vi "Get Control Refnum from Label.vi"(8 "error in (no error)":errorcluster, 9 "search field":enum16{"label", "caption", "label & caption"}(ring)=enum."label & caption", 10 "Control name":string, 11 "VI reference":refnum<vi>) -> (0 "error out":errorcluster, 1 "found?":bool, 2 "Ctl Refnum":refnum<vi>, 3 "VI reference out":refnum<vi>)   [LabVIEW 2009]
doc: "Takes a string and a reference to a VI, and searches all controls on the front panel of that VI for a control with a label that matches the input string, a label that does, or either one matches. Returns a reference to the first matching control found, or an empty reference if no controls matched."
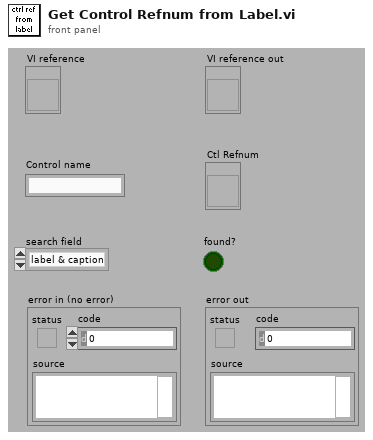
[diagram p1: front panel]
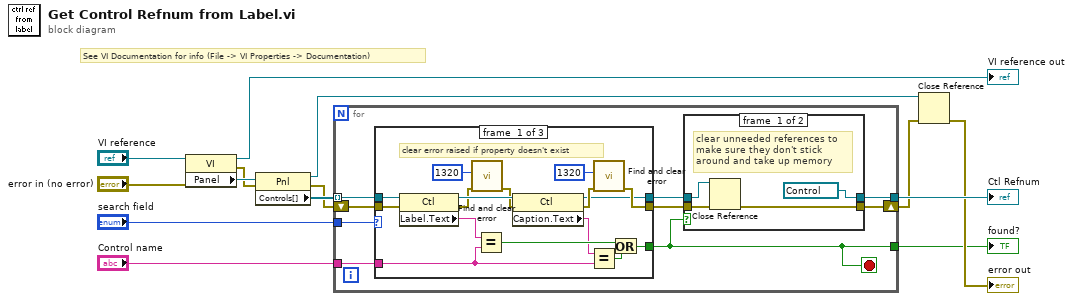
[diagram p0: block diagram]
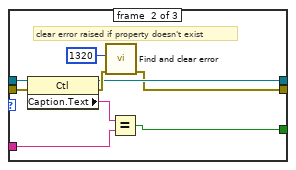
[diagram p2: hidden frame]
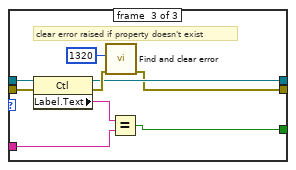
[diagram p3: hidden frame]
diagram:
  # "See VI Documentation for info (File -> VI Properties -> Documentation)"
  n1 = property class="VI"(reference="VI reference", error in="error in (no error)") -> (reference out=→"VI reference out":refnum<vi>, error out=w10:errorcluster, "Panel"=w13:refnum<vi>)
  n2 = property class="Pnl"(reference=w13, error in=w10) -> (reference out=w6:refnum<vi>, error out=w9:errorcluster, "Controls[]"=w12:refnum<vi>[])
  n3 = for {
    tunnel: w12 -> [w23] mode=indexing
    tunnel: "Control name" -> [w17]
    tunnel: [w15] -> w2
    shift-right: [w20] -> w5
    shift-left: w9 -> [w19]
    tunnel: [w18] -> w7
    tunnel: "search field" -> [w16]
    stop <- w15 stop-if-true
    n4 = case shown="\"label & caption\"" w16 {
      tunnel: w23 -> [w39 w48 w57]
      tunnel: [w27 w42 w51] -> w22
      tunnel: [w29 w41 w50] -> w21
      tunnel: w19 -> [w38 w47 w56]
      tunnel: w17 -> [w25 w43 w52]
      tunnel: [w35 w40 w49] -> w15
      frame #0 {
        # "clear error raised if property doesn't exist"
        n5 = property class="Ctl"(reference=w39, error in=w38) -> (reference out=w33:refnum<vi>, error out=w32:errorcluster, "Label.Text"=w37:string)
        n6 = call "Find and clear error.vi"("error in (no error)"=w32, "error code"=1320) -> ("error out"=w31:errorcluster)  [unwired: 9 out]
        n7 = Equal?(x=w37, y=w25) -> (x = y?=w36:bool)
        n8 = property class="Ctl"(reference=w33, error in=w31) -> (reference out=w27:refnum<vi>, error out=w28:errorcluster, "Caption.Text"=w26:string)
        n9 = Equal?(x=w26, y=w25) -> (x = y?=w24:bool)
        n10 = call "Find and clear error.vi"("error in (no error)"=w28, "error code"=1320) -> ("error out"=w29:errorcluster)  [unwired: 9 out]
        n11 = Or(x=w36, y=w24) -> (x .or. y?=w35:bool)
      }
      frame #1 {
        # "clear error raised if property doesn't exist"
        n12 = property class="Ctl"(reference=w48, error in=w47) -> (reference out=w42:refnum<vi>, error out=w44:errorcluster, "Caption.Text"=w46:string)
        n13 = call "Find and clear error.vi"("error in (no error)"=w44, "error code"=1320) -> ("error out"=w41:errorcluster)  [unwired: 9 out]
        n14 = Equal?(x=w46, y=w43) -> (x = y?=w40:bool)
      }
      frame #2 {
        # "clear error raised if property doesn't exist"
        n15 = property class="Ctl"(reference=w57, error in=w56) -> (reference out=w51:refnum<vi>, error out=w53:errorcluster, "Label.Text"=w55:string)
        n16 = call "Find and clear error.vi"("error in (no error)"=w53, "error code"=1320) -> ("error out"=w50:errorcluster)  [unwired: 9 out]
        n17 = Equal?(x=w55, y=w52) -> (x = y?=w49:bool)
      }
    }
    n18 = case shown="False" w15 {
      tunnel: w22 -> [w61 w62]
      tunnel: w21 -> [w60 w63]
      tunnel: [w59 w63] -> w20
      tunnel: [refnum<vi> refnum ("Ctl Refnum 2") w62] -> w18
      frame #0 {
        # "clear unneeded references to make sure they don't stick around and take up memory"
        n19 = Close Reference(reference=w61, error in (no error)=w60) -> (error out=w59:errorcluster)
      }
      frame #1 {
      }
    }
  }
  "Ctl Refnum" <- w7
  "found?" <- w2
  n20 = Close Reference(reference=w6, error in (no error)=w5) -> (error out=→"error out":errorcluster)
